vi "SetSensorData.vi"(4 "Sensor Data":T1) -> ()   [LabVIEW 2014]
uses:
  SensorData.ctl
  navXPacket.ctl
  EncoderPacket.ctl
  PotentiometerPacket.ctl
  distanceSensorPacket.ctl
  switchPacket.ctl
  SensorType.ctl
  SensorStatus.ctl
  Global Data.vi
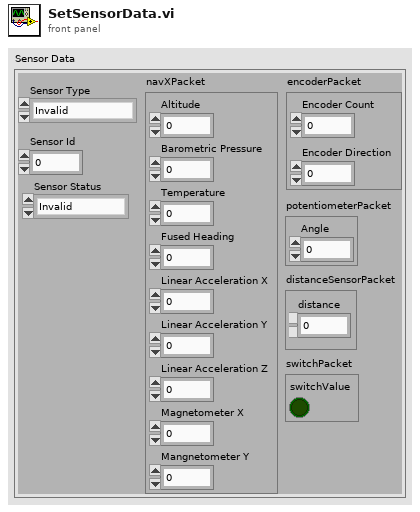
[diagram p1: front panel]
types:
  T1 = typedef "SensorData.ctl" = cluster{"Sensor Id":dbl, "navXPacket":T2, "encoderPacket":T3, "potentiometerPacket":T4, "distanceSensorPacket":T5, "switchPacket":T6, "Sensor Type":T7, "Sensor Status":T8}
  T2 = typedef "navXPacket.ctl" = cluster{"Altitude":dbl, "Barometric Pressure":dbl, "Fused Heading":dbl, "Linear Acceleration Y":dbl, "Linear Acceleration X":dbl, "Temperature":dbl, "Mangnetometer Y":dbl, "Magnetometer X":dbl, "Linear Acceleration Z":dbl}
  T3 = typedef "EncoderPacket.ctl" = cluster{"Encoder Count":dbl, "Encoder Direction":dbl}
  T4 = typedef "PotentiometerPacket.ctl" = cluster{"Angle":dbl}
  T5 = typedef "distanceSensorPacket.ctl" = cluster{"distance":dbl}
  T6 = typedef "switchPacket.ctl" = cluster{"switchValue":bool}
  T7 = typedef "SensorType.ctl" = enum16{"Invalid", "NavX", "Encoder", "Potentiometer", "Distance Sensor", "Switch"}
  T8 = typedef "SensorStatus.ctl" = enum16{"Invalid", "Operational", "Error occurred"}
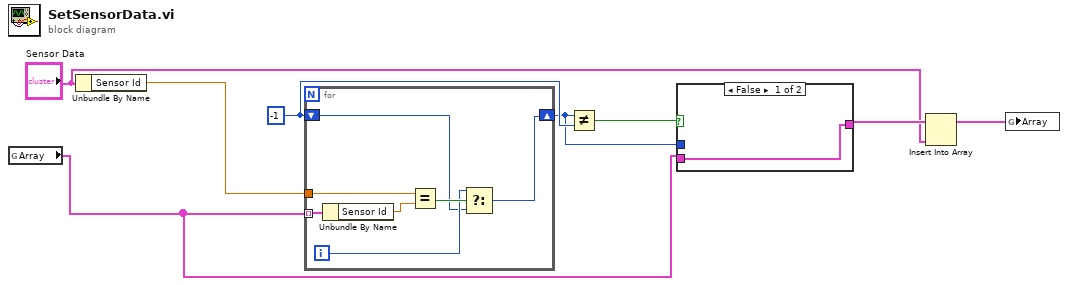
[diagram p0: block diagram]
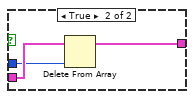
[diagram p2: hidden frame]
diagram:
  w7 = -1
  n1 = global read "Global Data.vi" "Array"() -> (w5:T1[])
  n2 = Unbundle By Name("Sensor Data") -> ("Sensor Id"=w8:dbl)
  n3 = for {
    tunnel: w5 -> [w15] mode=indexing
    shift-right: [w9] -> w4
    shift-left: w7 -> [w10]
    tunnel: w8 -> [w13]
    i -> [w11]
    n4 = Unbundle By Name(w15) -> ("Sensor Id"=w14:dbl)
    n5 = Equal?(x=w13, y=w14) -> (x = y?=w12:bool)
    n6 = Select(t=w11, s=w12, f=w10) -> (s? t:f=w9:i32)
  }
  n7 = Not Equal?(x=w4, y=w7) -> (x != y?=w6:bool)
  n8 = case shown="False" w6 {
    tunnel: w5 -> [w16 w19]
    tunnel: w4 -> [_ w18]
    tunnel: [w16 w17] -> w3
    frame False {
    }
    frame True {
      n9 = Delete From Array(array=w19, index=w18) -> (array with subset deleted=w17:T1[])  [unwired: 1 in, 1 out]
    }
  }
  n10 = Insert Into Array(array=w3, new element="Sensor Data") -> (w1:T1[])  [unwired: 1 in]
  n11 = global write "Global Data.vi" "Array"(w1) -> ()
